vi "Li_execfun_svi.vi"(7 "OP":T1=enum."Push", 8 "error in (no error)":errorcluster, 10 "Key Index":i32, 11 "IN":i32) -> (0 "error out":errorcluster, 2 "Size":i32, 3 "Addr":i32)   [LabVIEW 2015]
uses:
  LIFO.ctl
  C:/Users/Giuseppe/Downloads/LabLinda_ pakage/index_datatype.ctl
  C:/Users/Giuseppe/Downloads/LabLinda_ pakage/index_cluster.ctl
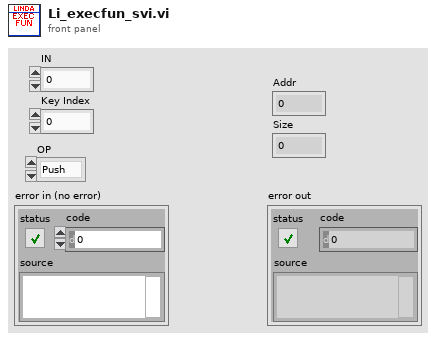
[diagram p1: front panel]
types:
  T1 = typedef "LIFO.ctl" = enum16{"INIT", "Push", "Pop", "Query", "BPush"}
  T2 = typedef "index_datatype.ctl" = T3[]
  T3 = typedef "index_cluster.ctl" = cluster{"Addr":i32[], "out react vi reference":refnum<vi>, "in react vi reference":refnum<vi>, "rd react vi reference":refnum<vi>, "Read_write_var":refnum<vi>}
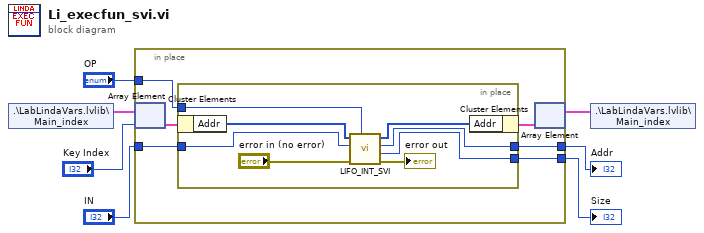
[diagram p0: block diagram]
diagram:
  n1 = shared-variable ".\\LabLindaVars.lvlib\\Main_index"() -> (w2:T2)  [unwired: 1 in, 1 out]
  n2 = in-place {
    in-place-border: [w13] -> w5
    in-place-border: [w12] -> w4
    in-place-border: "OP" -> [w11]
    in-place-border: "IN" -> [w10]
    n3 = in-place-array #1(w2, "Key Index") -> (w8:T3)
    n4 = in-place {
      in-place-border: [w20] -> w13
      in-place-border: [w19] -> w12
      in-place-border: w11 -> [w18]
      in-place-border: w10 -> [w17]
      n5 = in-place-cluster #2(w8) -> ("Addr"=w14:i32[])
      n6 = call "LIFO_INT_SVI.vi"("OP"=w18, "error in (no error)"="error in (no error)", "IN"=w17, "Array IN"=w14) -> ("error out"=→"error out":errorcluster, "Size"=w20:i32, "Elem"=w19:i32, "Array"=w21:i32[])  [unwired: 4 in]
      n7 = in-place-cluster #2("Addr"=w21) -> (w9:T3)
    }
    n8 = in-place-array #1(w9) -> (w1:T2)  [unwired: 1 out]
  }
  "Addr" <- w4
  "Size" <- w5
  n9 = shared-variable ".\\LabLindaVars.lvlib\\Main_index"(w1) -> ()  [unwired: 1 in, 1 out]
